vi "Example - Label.vi"() -> ()   [LabVIEW 2020]
uses:
  Label Properties.ctl
  Font Style.ctl
  Dot Net UI Controls.lvlib
  System.Windows.Forms
panel:
  in  "Properties":T1={"Font Name"="Segoe UI", "Size"=20.0, "Style"=enum."Underline", "Align"=32, "FG Color"=16777215, "BG Color"=16229888} {"Align" items=["TopLeft"=1, "TopCenter"=2, "TopRight"=4, "MiddleLeft"=16, "MiddleCenter"=32, "MiddleRight"=64, "BottomLeft"=256, "BottomCenter"=512, "BottomRight"=1024]}
  in  "Text":string="Hello World!"
  in  "Stop":bool
  in  "Label":refnum<k24>(container)
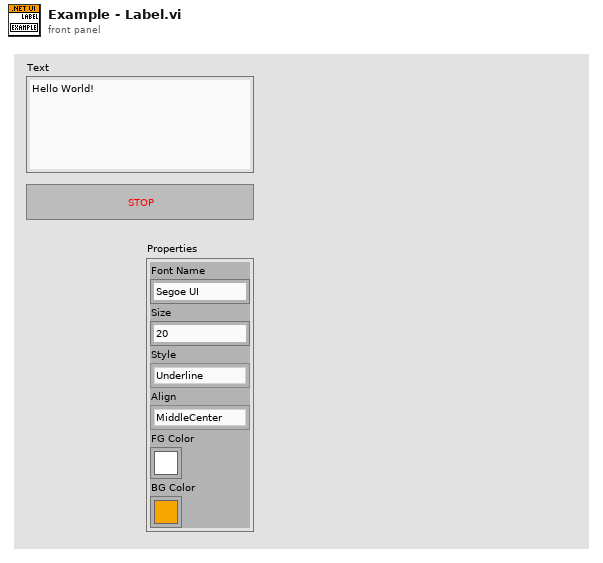
[diagram p1: front panel]
types:
  T1 = typedef "Dot Net UI Controls.lvlib/Label Properties.ctl" = cluster{"Font Name":string, "Size":sgl, "Style":T2, "Align":i32, "FG Color":u32, "BG Color":u32}
  T2 = typedef "Dot Net UI Controls.lvlib/Font Style.ctl" = enum16{"Regular", "Bold", "Italic", "Underline", "Strikeout"}
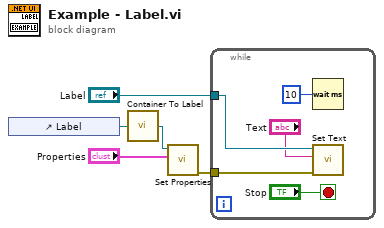
[diagram p0: block diagram]
diagram:
  n1 = control-ref of="Label"() -> (w2:refnum<vi>)
  n2 = call "Container To Label.vi"("ActiveX Container"=w2) -> ("Label"=w1:refnum<k24>)
  n3 = call "Set Properties.vi"("Properties"="Properties", "Label In"=w1) -> ("Error Out"=w5:errorcluster)  [unwired: 8 in, 1 out]
  n4 = while {
    tunnel: w5 -> [w6]
    tunnel: "Label" -> [w10]
    stop <- "Stop" stop-if-true
    n5 = Wait (ms)(milliseconds to wait=u32 10) -> ()  [unwired: 1 out]
    n6 = call "Set Text.vi"("Error In"=w6, "Text"="Text", "Label In"=w10) -> ()  [unwired: 7 in, 2 out]
  }
